vi "Maxi Gauge Terminator -- Point.vi"(1 "Eingangstring":string="  0F 400  EE2") -> (0 "Ausgangstring":string="03")   [LabVIEW 2012, in "Maxi Gauge.lvlib"]
uses:
  Maxi Gauge.lvlib
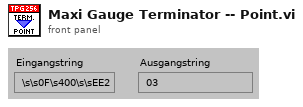
[diagram p1: front panel]
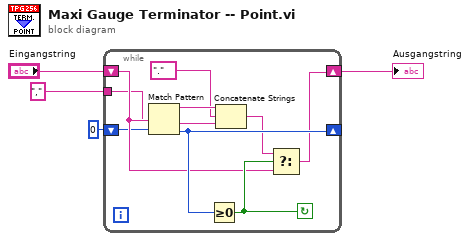
[diagram p0: block diagram]
diagram:
  n1 = while {
    tunnel: "," ("Terminator") -> [w6]
    shift-left: "Eingangstring" -> [w9]
    shift-right: [w8] -> w3
    shift-left: 0 -> [w7]
    shift-right: [w12] -> _
    stop <- w10 continue-if-true
    n2 = Match Pattern(string=w9, regular expression=w6, offset (0)=w7) -> (before substring=w14:string, after substring=w13:string, offset past match=w12:i32)  [unwired: 1 out]
    n3 = Greater Or Equal To 0?(x=w12) -> (x >= 0?=w10:bool)
    n4 = Concatenate Strings(w14, ".", w13) -> (w11:string)
    n5 = Select(t=w11, s=w10, f=w9) -> (s? t:f=w8:string)
  }
  "Ausgangstring" <- w3
